vi "Move DC_X_Distance.vi"   [LabVIEW 2012, in "4134Outputs.lvlib"]
uses:
  4134Outputs.lvlib
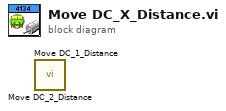
[diagram p0: block diagram]
diagram:
  n1 = call "Move DC_2_Distance.vi"() -> ()  [unwired: 15 in, 1 out]
  n2 = call "Move DC_1_Distance.vi"() -> ()  [unwired: 15 in, 1 out]
